vi "Do.vi"(8 "error in":errorcluster, 10 "Actor in":refnum<class "Actor.lvclass">, 11 "Send New Setpoint":refnum<class "Send New Setpoint.lvclass">) -> (0 "error out":errorcluster, 2 "Actor out":refnum<class "Actor.lvclass">)   [LabVIEW 2015]
doc: "(<B>Filename</B>: Actor Framework.lvlib:Message.lvclass:Do.vi)\n\nDefines what a message does when it is received by an actor. Generally, a message instructs an actor to invoke one of its methods. By default, this method does nothing. A child class must override it to define behavior. Create a child class by using the Actor Framework Message Maker dialog box."
uses:
  reusable/DAQ Device/Device/Device.lvclass
  reusable/Session APIs/CVT/CVT.lvclass
  Configurable Device.lvclass
  <vilib>/ActorFramework/Actor/Actor.lvclass
  Send New Setpoint.lvclass
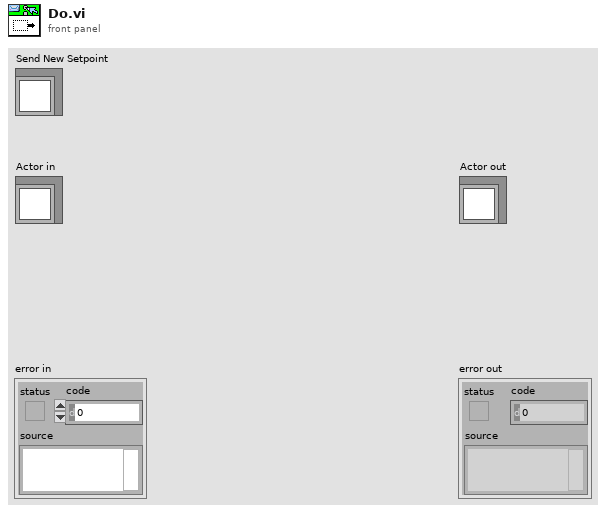
[diagram p1: front panel]
types:
  T1 = typedef "Session - Root.lvclass/Session Handle.ctl" = refnum<data-value>
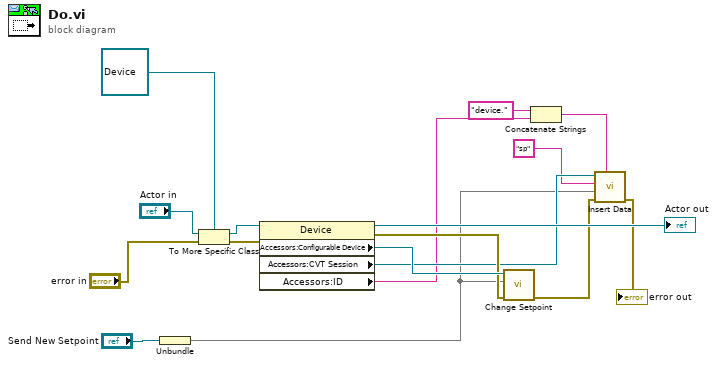
[diagram p0: block diagram]
diagram:
  n1 = Unbundle("Send New Setpoint") -> (w1)
  n2 = To More Specific Class(target class=refnum<class "Device.lvclass"> refnum ("DAQ Device.lvlib:Device"), reference="Actor in", error in="error in") -> (specific class reference=w14:refnum<class "Device.lvclass">, error out=w13:errorcluster)
  n3 = property class="Device"(reference=w14, error in=w13) -> (reference out=→"Actor out":refnum<class "Device.lvclass">, error out=w9:errorcluster, "Accessors:Configurable Device"=w10:refnum<class "Configurable Device.lvclass">, "Accessors:CVT Session"=w8:T1, "Accessors:ID"=w5:string)
  n4 = call-dynamic "Change Setpoint.vi"("error in (no error)"=w9, "Setpoint"=w1, "Configurable Device in"=w10) -> ("error out"=w7:errorcluster)  [unwired: 7 in, 1 out]
  n5 = Concatenate Strings("device." ("string"), w5) -> (w3:string)
  n6 = call "Insert Data.vi"("Group"=w3, "error in"=w7, "Data"=w1, "tag"="sp", "CVT Session In"=w8) -> ("error out"=→"error out":errorcluster)  [unwired: 5 in, 1 out]
